vi "Elevator Config.vi"(8 "error in (no error)":errorcluster, 11 "FileConfig in":refnum<class "FileConfig.lvclass">) -> (0 "error out":errorcluster, 1 "IDs found?":bool, 2 "Elevator Data":T1={"Wrist"=0, "Left Master"=0, "Left Slave"=0, "Right Master"=0, "Right Slave"=0, "Elevator Wrist PID"={"P"=0.0, "I"=0.0, "D"=0.0, "F"=0.0, "integralZone"=0.0, "allowableClosedLoopError"=0, "maxIntegralAccumulator"=0.0, "closedLoopPeakOutput"=1.0, "closedLoopPeriod"=1}, "Elevator Arm PID"={"P"=0.0, "I"=0.0, "D"=0.0, "F"=0.0, "integralZone"=0.0, "allowableClosedLoopError"=0, "maxIntegralAccumulator"=0.0, "closedLoopPeakOutput"=1.0, "closedLoopPeriod"=1}, "Vacumm Pump 1"=0, "Vacumm Pump 2"=0, "Arm Motion Magic Max Velocity"=0, "Arm Motion Magic Max Acceleration"=0, "Wrist Motion Magic Max Velocity"=0, "Wrist Motion Magic Max Acceleration"=0, "Arm Gear Ratio"=0.0, "Wrist Gear Ratio"=0.0, "C0 Arm"=0.0, "C1 Arm"=0.0, "C2 Arm"=0.0, "H1 Arm"=0.0, "H2 Arm"=0.0, "C0 Wrist"=0.0, "C1 Wrist "=0.0, "C2 Wrist"=0.0, "H1 Wrist"=0.0, "H2 Wrist"=0.0, "Deploy Arm"=0.0, "Deploy Wrist"=0.0, "Climb Arm"=0.0, "Climb Wrist"=0.0, "Arm Encoder ABS Value"=0, "Wrist Encoder ABS Value"=0}, 3 "FileConfig out":refnum<class "FileConfig.lvclass">, 4 "PIDFs found":bool, 5 "File Found?":bool)   [LabVIEW 2018, in "Config.lvlib" / "FileConfig.lvclass"]
doc: "Use this VI to get the configuration for the Elevator CAN IDs"
uses:
  FileConfig.lvclass
  Config/Controls/Elevator Data.ctl
  <vilib>/Rock Robotics/WPI/ThirdParty/Phoenix-LabVIEW/Motor Controller/Controls/CTRE_Phoenix_MotorControl_SlotStructure.ctl
  FileConfig.lvclass/FileConfig.ctl
  Config.lvclass
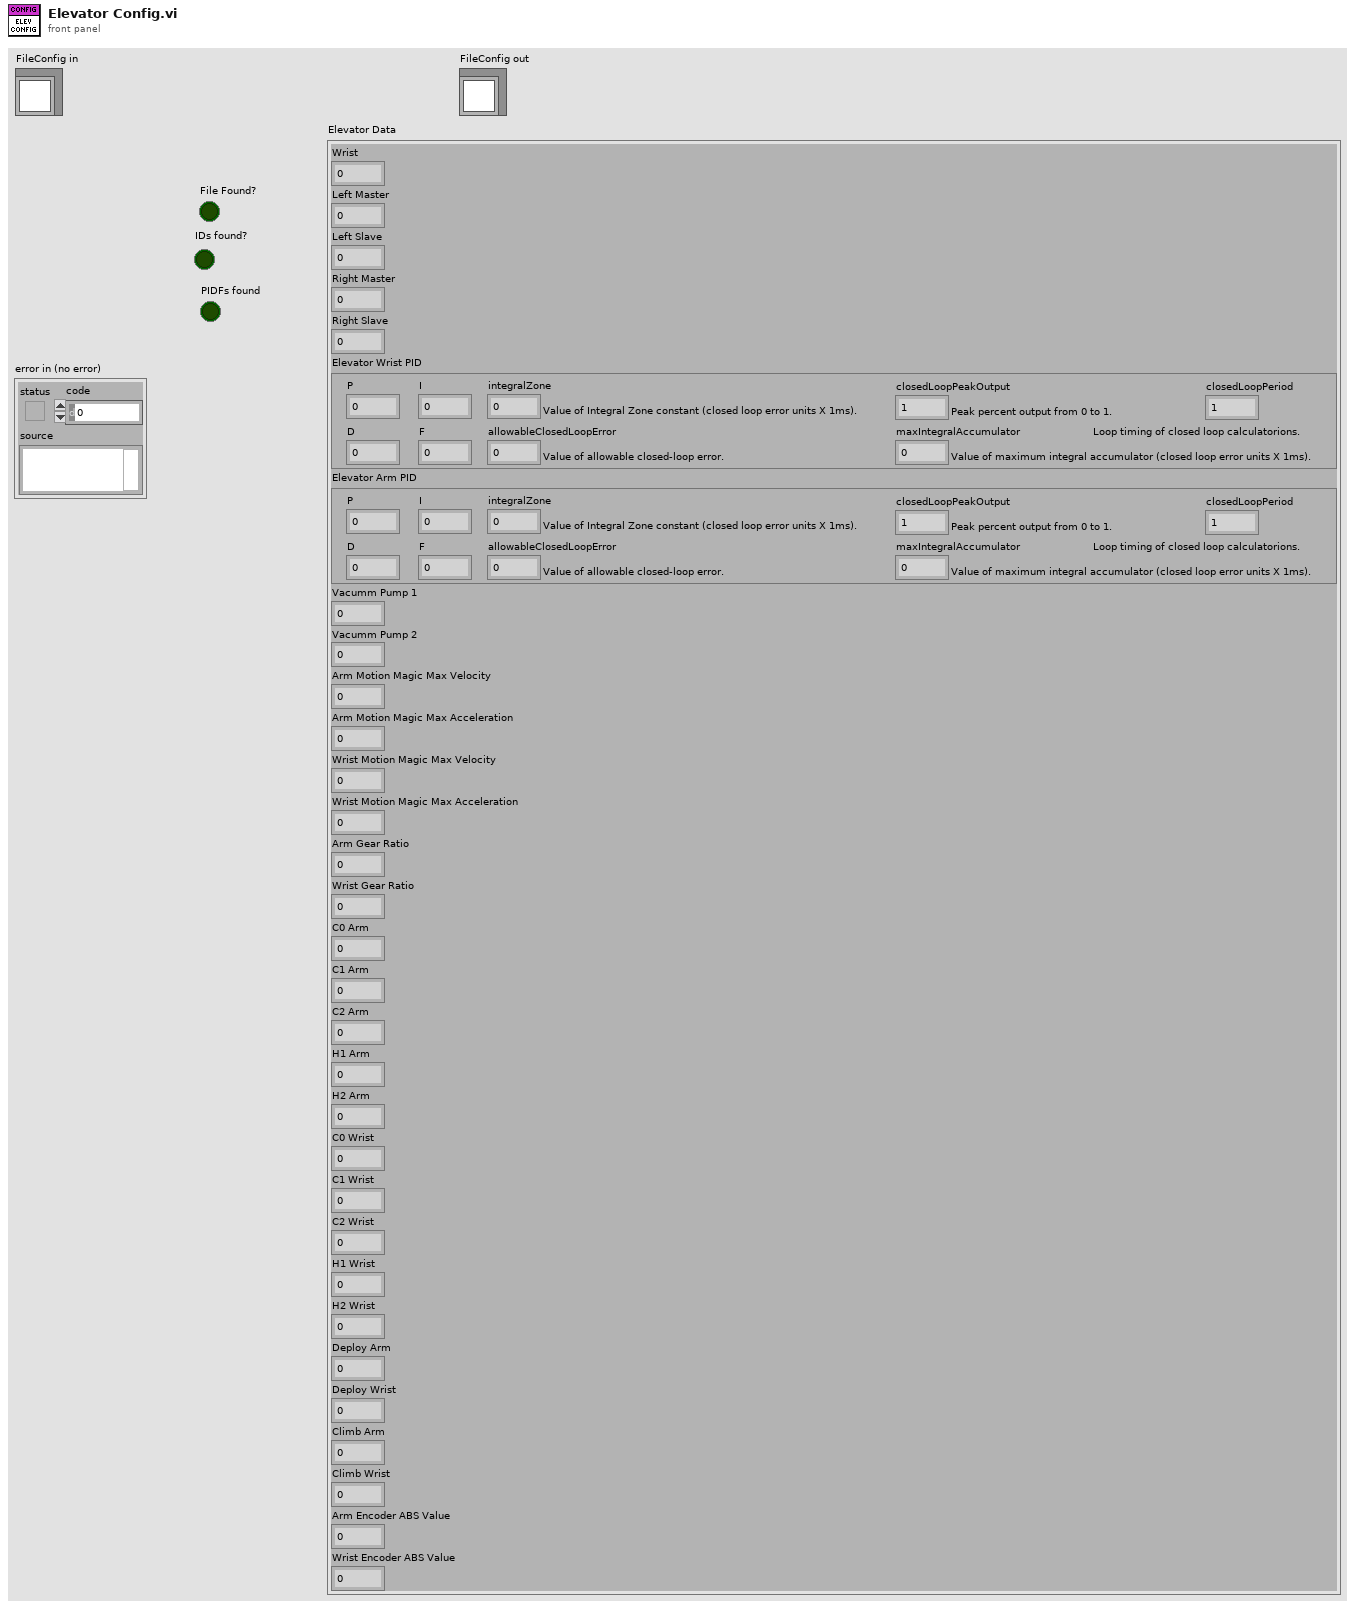
[diagram p1: front panel]
types:
  T1 = typedef "Config.lvlib/Config.lvclass/Elevator Data.ctl" = cluster{"Wrist":u8, "Left Master":u8, "Left Slave":u8, "Right Master":u8, "Right Slave":u8, "Elevator Wrist PID":T2, "Elevator Arm PID":T2, "Vacumm Pump 1":u8, "Vacumm Pump 2":u8, "Arm Motion Magic Max Velocity":u32, "Arm Motion Magic Max Acceleration":u32, "Wrist Motion Magic Max Velocity":u32, "Wrist Motion Magic Max Acceleration":u32, "Arm Gear Ratio":dbl, "Wrist Gear Ratio":dbl, "C0 Arm":dbl, "C1 Arm":dbl, "C2 Arm":dbl, "H1 Arm":dbl, "H2 Arm":dbl, "C0 Wrist":dbl, "C1 Wrist ":dbl, "C2 Wrist":dbl, "H1 Wrist":dbl, "H2 Wrist":dbl, "Deploy Arm":dbl, "Deploy Wrist":dbl, "Climb Arm":dbl, "Climb Wrist":dbl, "Arm Encoder ABS Value":i32, "Wrist Encoder ABS Value":i32}
  T2 = typedef "CTRE_Phoenix_MotorControl_SlotStructure.ctl" = cluster{"P":dbl, "I":dbl, "D":dbl, "F":dbl, "integralZone":dbl, "allowableClosedLoopError":i32, "maxIntegralAccumulator":dbl, "closedLoopPeakOutput":dbl, "closedLoopPeriod":i32}
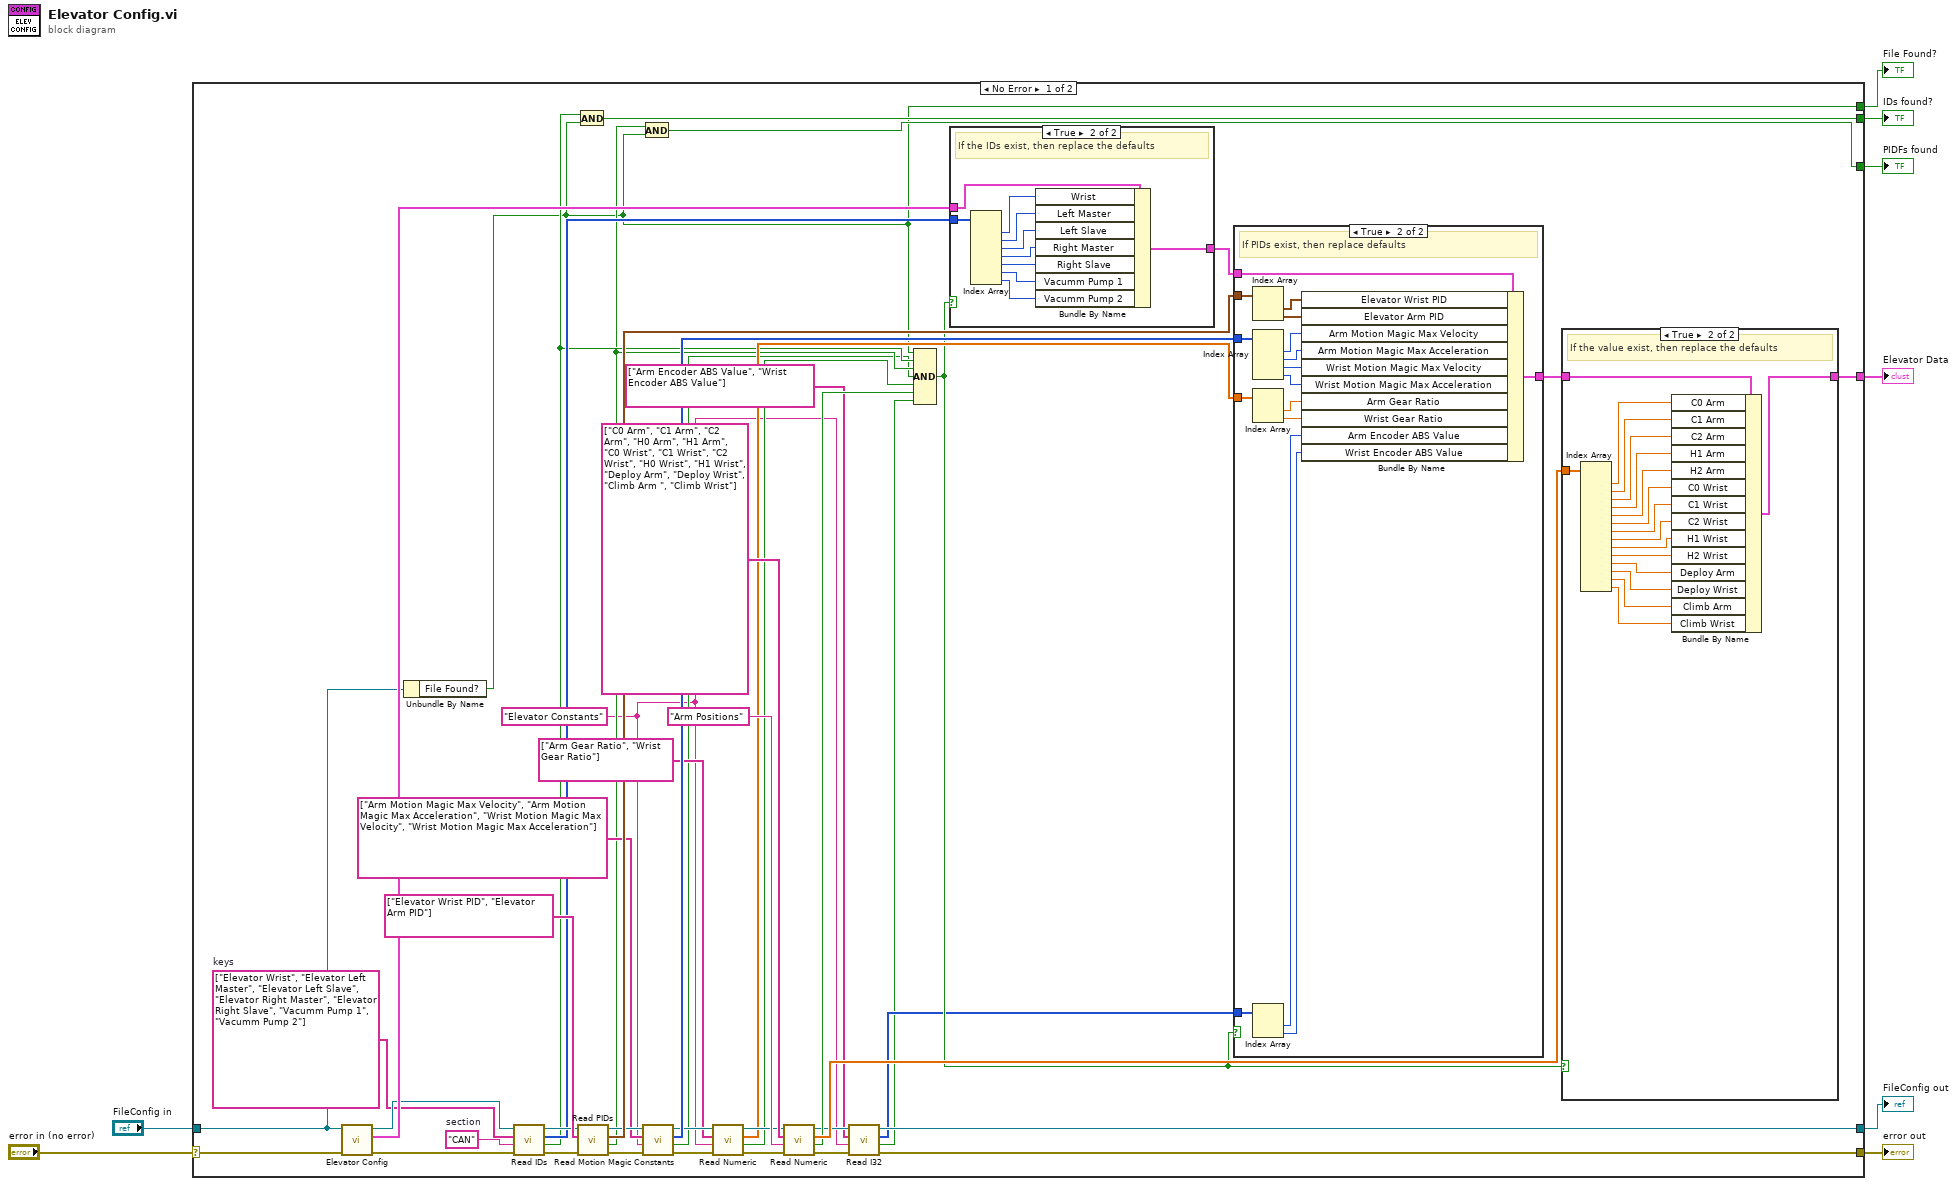
[diagram p0: block diagram]
diagram:
  n1 = case shown="No Error" "error in (no error)" {
    selector: "error in (no error)" -> [w51 w100]
    tunnel: "FileConfig in" -> [w52 w101]
    tunnel: [w13 w100] -> w6
    tunnel: [w34 _] -> w5
    tunnel: [w15 w101] -> w4
    tunnel: [w18 _] -> w3
    tunnel: [w25 _] -> w2
    tunnel: [w24 _] -> w1
    frame No Error {
      w10 = "Elevator Constants" ("section")
      w45 = string[] ["Elevator Wrist", "Elevator Left Master", "Elevator Left Slave", "Elevator Right Master", "Elevator Right Slave", "Vacumm Pump 1", "Vacumm Pump 2"]  # keys
      w44 = "CAN"  # section
      n2 = call-parent "Elevator Config.vi"("error in (no error)"=w51, "Config in"=w52) -> ("error out"=w46:errorcluster, "Elevator Data"=w53:T1, "Config out"=w47:refnum<class "FileConfig.lvclass">)  [unwired: 4 in, 3 out]
      n3 = Unbundle By Name(w52) -> ("File Found?"=w18:bool)
      n4 = call "Read IDs.vi"("error in (no error)"=w46, "section"=w44, "keys"=w45, "FileConfig in"=w47) -> ("error out"=w42:errorcluster, "Found?"=w23:bool, "Found IDs"=w41:u8[], "FileConfig out"=w43:refnum<class "FileConfig.lvclass">)  [unwired: 4 in]
      n5 = And(x=w23, y=w18) -> (x .and. y?=w25:bool)
      n6 = call "Read PIDs.vi"("error in (no error)"=w42, "PID Sections to read"=string[] ["Elevator Wrist PID", "Elevator Arm PID"], "FileConfig in"=w43) -> ("error out"=w38:errorcluster, "Found?"=w22:bool, "PIDF Array"=w50:T2[], "FileConfig out"=w40:refnum<class "FileConfig.lvclass">)  [unwired: 5 in]
      n7 = And(x=w22, y=w18) -> (x .and. y?=w24:bool)
      n8 = call "Read Motion Magic Constants.vi"("error in (no error)"=w38, "section"=w10, "keys"=string[] ["Arm Motion Magic Max Velocity", "Arm Motion Magic Max Acceleration", "Wrist Motion Magic Max Velocity", "Wrist Motion Magic Max Acceleration"] ("PID Sections to read"), "FileConfig in"=w40) -> ("error out"=w29:errorcluster, "Found?"=w21:bool, "Found Constants"=w37:u32[], "FileConfig out"=w31:refnum<class "FileConfig.lvclass">)  [unwired: 4 in]
      n9 = call "Read Numeric.vi"("error in (no error)"=w29, "section"=w10, "keys"=string[] ["Arm Gear Ratio", "Wrist Gear Ratio"], "FileConfig in"=w31) -> ("error out"=w28:errorcluster, "Found?"=w20:bool, "Found DBL"=w26:dbl[], "FileConfig out"=w30:refnum<class "FileConfig.lvclass">)  [unwired: 4 in]
      n10 = call "Read Numeric.vi"("error in (no error)"=w28, "section"="Arm Positions", "keys"=string[] ["C0 Arm", "C1 Arm", "C2 Arm", "H0 Arm", "H1 Arm", "C0 Wrist", "C1 Wrist", "C2 Wrist", "H0 Wrist", "H1 Wrist", "Deploy Arm", "Deploy Wrist", "Climb Arm ", "Climb Wrist"], "FileConfig in"=w30) -> ("error out"=w14:errorcluster, "Found?"=w19:bool, "Found DBL"=w36:dbl[], "FileConfig out"=w16:refnum<class "FileConfig.lvclass">)  [unwired: 4 in]
      n11 = call "Read I32.vi"("error in (no error)"=w14, "section"=w10, "keys"=string[] ["Arm Encoder ABS Value", "Wrist Encoder ABS Value"], "FileConfig in"=w16) -> ("error out"=w13:errorcluster, "Found?"=w9:bool, "Found I32"=w11:i32[], "FileConfig out"=w15:refnum<class "FileConfig.lvclass">)  [unwired: 4 in]
      n12 = Compound Arithmetic op=AND(w18, w23, w22, w21, w20, w19, w9) -> (w17:bool)
      n13 = case shown="True" w17 {
        tunnel: w53 -> [w89 w99]
        tunnel: [w89 w98] -> w49
        tunnel: w41 -> [_ w97]
        frame False {
        }
        frame True {
          # "If the IDs exist, then replace the defaults"
          n14 = Index Array(array=w97) -> (element #1=w93:u8, element #2=w96:u8, element #3=w95:u8, element #4=w94:u8, element #5=w92:u8, element #6=w91:u8, element #7=w90:u8)  [unwired: 7 in]
          n15 = Bundle By Name(cluster=w99, "Wrist"=w93, "Left Master"=w96, "Left Slave"=w95, "Right Master"=w94, "Right Slave"=w92, "Vacumm Pump 1"=w91, "Vacumm Pump 2"=w90) -> (w98:T1)
        }
      }
      n16 = case shown="True" w17 {
        tunnel: w49 -> [w72 w88]
        tunnel: [w72 w87] -> w35
        tunnel: w50 -> [_ w86]
        tunnel: w37 -> [_ w83]
        tunnel: w26 -> [_ w78]
        tunnel: w11 -> [_ w75]
        frame False {
        }
        frame True {
          # "If PIDs exist, then replace defaults"
          n17 = Index Array(array=w86) -> (element #1=w85:T2, element #2=w84:T2)  [unwired: 2 in]
          n18 = Index Array(array=w83) -> (element #1=w82:u32, element #2=w81:u32, element #3=w80:u32, element #4=w79:u32)  [unwired: 4 in]
          n19 = Index Array(array=w78) -> (element #1=w77:dbl, element #2=w76:dbl)  [unwired: 2 in]
          n20 = Index Array(array=w75) -> (element #1=w74:i32, element #2=w73:i32)  [unwired: 2 in]
          n21 = Bundle By Name(cluster=w88, "Elevator Wrist PID"=w85, "Elevator Arm PID"=w84, "Arm Motion Magic Max Velocity"=w82, "Arm Motion Magic Max Acceleration"=w81, "Wrist Motion Magic Max Velocity"=w80, "Wrist Motion Magic Max Acceleration"=w79, "Arm Gear Ratio"=w77, "Wrist Gear Ratio"=w76, "Arm Encoder ABS Value"=w74, "Wrist Encoder ABS Value"=w73) -> (w87:T1)
        }
      }
      n22 = case shown="True" w17 {
        tunnel: w35 -> [w54 w71]
        tunnel: [w54 w70] -> w34
        tunnel: w36 -> [_ w69]
        frame False {
        }
        frame True {
          # "If the value exist, then replace the defaults"
          n23 = Index Array(array=w69) -> (element #1=w68:dbl, element #2=w67:dbl, element #3=w66:dbl, element #4=w65:dbl, element #5=w64:dbl, element #6=w63:dbl, element #7=w62:dbl, element #8=w61:dbl, element #9=w60:dbl, element #10=w59:dbl, element #11=w58:dbl, element #12=w57:dbl, element #13=w56:dbl, element #14=w55:dbl)  [unwired: 14 in]
          n24 = Bundle By Name(cluster=w71, "C0 Arm"=w68, "C1 Arm"=w67, "C2 Arm"=w66, "H1 Arm"=w65, "H2 Arm"=w64, "C0 Wrist"=w63, "C1 Wrist"=w62, "C2 Wrist"=w61, "H1 Wrist"=w60, "H2 Wrist"=w59, "Deploy Arm"=w58, "Deploy Wrist"=w57, "Climb Arm"=w56, "Climb Wrist"=w55) -> (w70:T1)
        }
      }
    }
    frame Error {
    }
  }
  "error out" <- w6
  "FileConfig out" <- w4
  "File Found?" <- w3
  "IDs found?" <- w2
  "Elevator Data" <- w5
  "PIDFs found" <- w1
